vi "一体站流程自动启动.vi"(11 "参数":T1) -> ()   [LabVIEW 2016, in "PLC.lvlib"]
uses:
  PLC.lvlib
  <vilib>/ptbypt/NI_PtbyPt.lvlib
panel:
  out "s? t:f":enum16{"初始化", "采配水启动", "仪器操作", "反冲洗", "结束"}(ring)
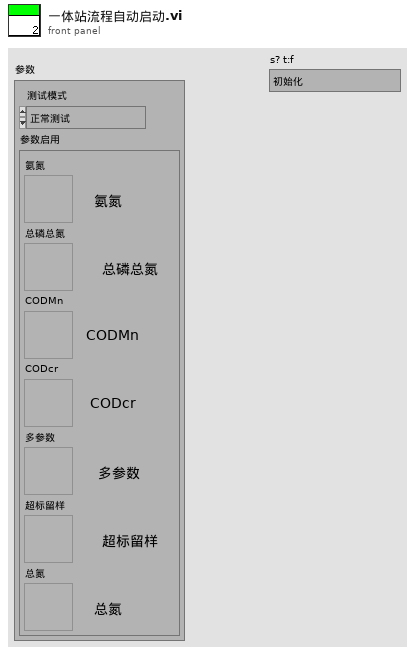
[diagram p1: front panel]
types:
  T1 = cluster{"测试模式":enum16{"正常测试", "集成干预"}, "参数启用":cluster{"氨氮":bool, "总磷总氮":bool, "CODMn":bool, "CODcr":bool, "多参数":bool, "超标留样":bool, "总氮":bool}}
  T2 = cluster{"命令":string, cluster{"starting address":u16, "holding register value":u16}}
  T3 = enum16{"加标流程（润洗/采样分开）", "加标流程（润洗/采样合并）", "加标流程（不启动采配水）", "水样测试（润洗/采样分开）", "水样测试（润洗/采样合并）", "水样测试（不启动采配水）"}
  T4 = typedef "质控单元V4.lvlib/质控slave id.ctl" = enum16{"null", "氨氮", "总磷", "总氮", "CODMn", "CODCr", "氨氮总磷", "总磷总氮"}
  T5 = cluster{"时间标识":timestamp, "设备":string, "日志信息":string, "流程参数":string}
  T6 = cluster{"测量模式":enum16{"水样测量", "标样核查", "零点核查", "跨度核查", "空白测试", "加标回收", "平行样", "校零", "校标"}}
  T7 = cluster{"时间标识":timestamp, "设备":string, "日志信息":string}
  T8 = enum16{"空闲", "水样测试", "标样核查", "零点核查", "跨度核查", "空白测试", "平行样测试", "加标回收", "空白校准", "标样校准", "初始化（清洗）"}
  T9 = enum32{"Bad", "Idle", "Run top level", "Running"}
  T10 = cluster{"R0":i16, "R1":i16, "R2":i16, "R3":i16, "R4":i16, "R5":i16, "R6":i16, "R7":i16, "R8":i16, "R9":i16, "R10":i16, "R11":i16, "R12":i16, "R13":i16, "R14":i16, "R15":i16, "R16":i16, "R17":i16, "R18":i16, "R19":i16, "R20":i16, "R21":i16, "R22":i16, "R23":i16, "R24":i16, "R25":i16, "R26":i16, "R27":i16, "R28":i16, "R29":i16, "R30":i16, "R31":i16, "R32":i16, "R33":i16, "R34":i16, "R35":i16, "R36":i16, "R37":i16, "R38":i16, "R39":i16, "R40":i16, "R41":i16, "R42":i16, "R43":i16, "R44":i16, "R45":i16, "R46":i16, "R47":i16, "R48":i16, "R49":i16, "R50":i16, "R51":i16, "R52":i16, "R53":i16, "R54":i16, "R55":i16, "R56":i16}
  T11 = cluster{"氨氮":bool, "总磷总氮":bool, "CODmn":bool, "CODCr":bool, "多参数":bool, "超标留样":bool, "总氮":bool}
  T12 = cluster{"因子编码":u32, "单位":u16, "标样参考值":sgl, "水样数据时间":timestamp, "水样实测值":sgl, "水样数据标识":string, "标样数据时间":timestamp, "标样实测值":sgl, "标样数据标识":string, "空白数据时间":timestamp, "空白实测值":sgl, "空白数据标识":string, "零点核查数据时间":timestamp, "零点核查实测值":sgl, "零点核查数据标识":string, "跨度核查数据时间":timestamp, "跨度核查实测值":sgl, "跨度核查数据标识":string, "加标回收数据时间":timestamp, "加标回收实测值":sgl, "加标回收数据标识":string, "平行样数据时间":timestamp, "平行样实测值":sgl, "平行样数据标识":string, "F0":sgl, "F1":sgl, "F2":sgl, "F3":sgl, "F4":sgl, "F5":sgl, "F6":sgl, "F7":sgl, "温度":sgl, "湿度":sgl, "X值":sgl, "fidrange":u16}
  T13 = cluster{"COD浓度（mg/L)":dbl, "水样启动时间":timestamp, "加标回收启动时间":timestamp, "CODMn工作状态":enum16{"空闲", "水样测试", "标样核查", "零点核查", "跨度核查", "空白测试", "平行样测试", "加标回收", "空白校准", "标样校准", "初始化（清洗）"}, "多列列表框":i32}
  T14 = cluster{"因子编码":u32, "单位":u16, "标样参考值":sgl, "水样数据时间":timestamp, "水样实测值":sgl, "水样数据标识":string, "标样数据时间":timestamp, "标样实测值":sgl, "标样数据标识":string, "空白数据时间":timestamp, "空白实测值":sgl, "空白数据标识":string, "零点核查数据时间":timestamp, "零点核查实测值":sgl, "零点核查数据标识":string, "跨度核查数据时间":timestamp, "跨度核查实测值":sgl, "跨度核查数据标识":string, "加标回收数据时间":timestamp, "加标回收实测值":sgl, "加标回收数据标识":string, "平行样数据时间":timestamp, "平行样实测值":sgl, "平行样数据标识":string}
  T15 = cluster{"氨氮":bool, "总磷总氮":bool, "CODMn":bool, "CODcr":bool, "多参数":bool, "超标留样":bool, "总氮":bool}
  T16 = cluster{"时间标识":timestamp, "参数":string, "数据类型":string, "集成干预测试浓度值":dbl, "集成干预前测试时间":timestamp, "集成干预前测试浓度值":dbl}
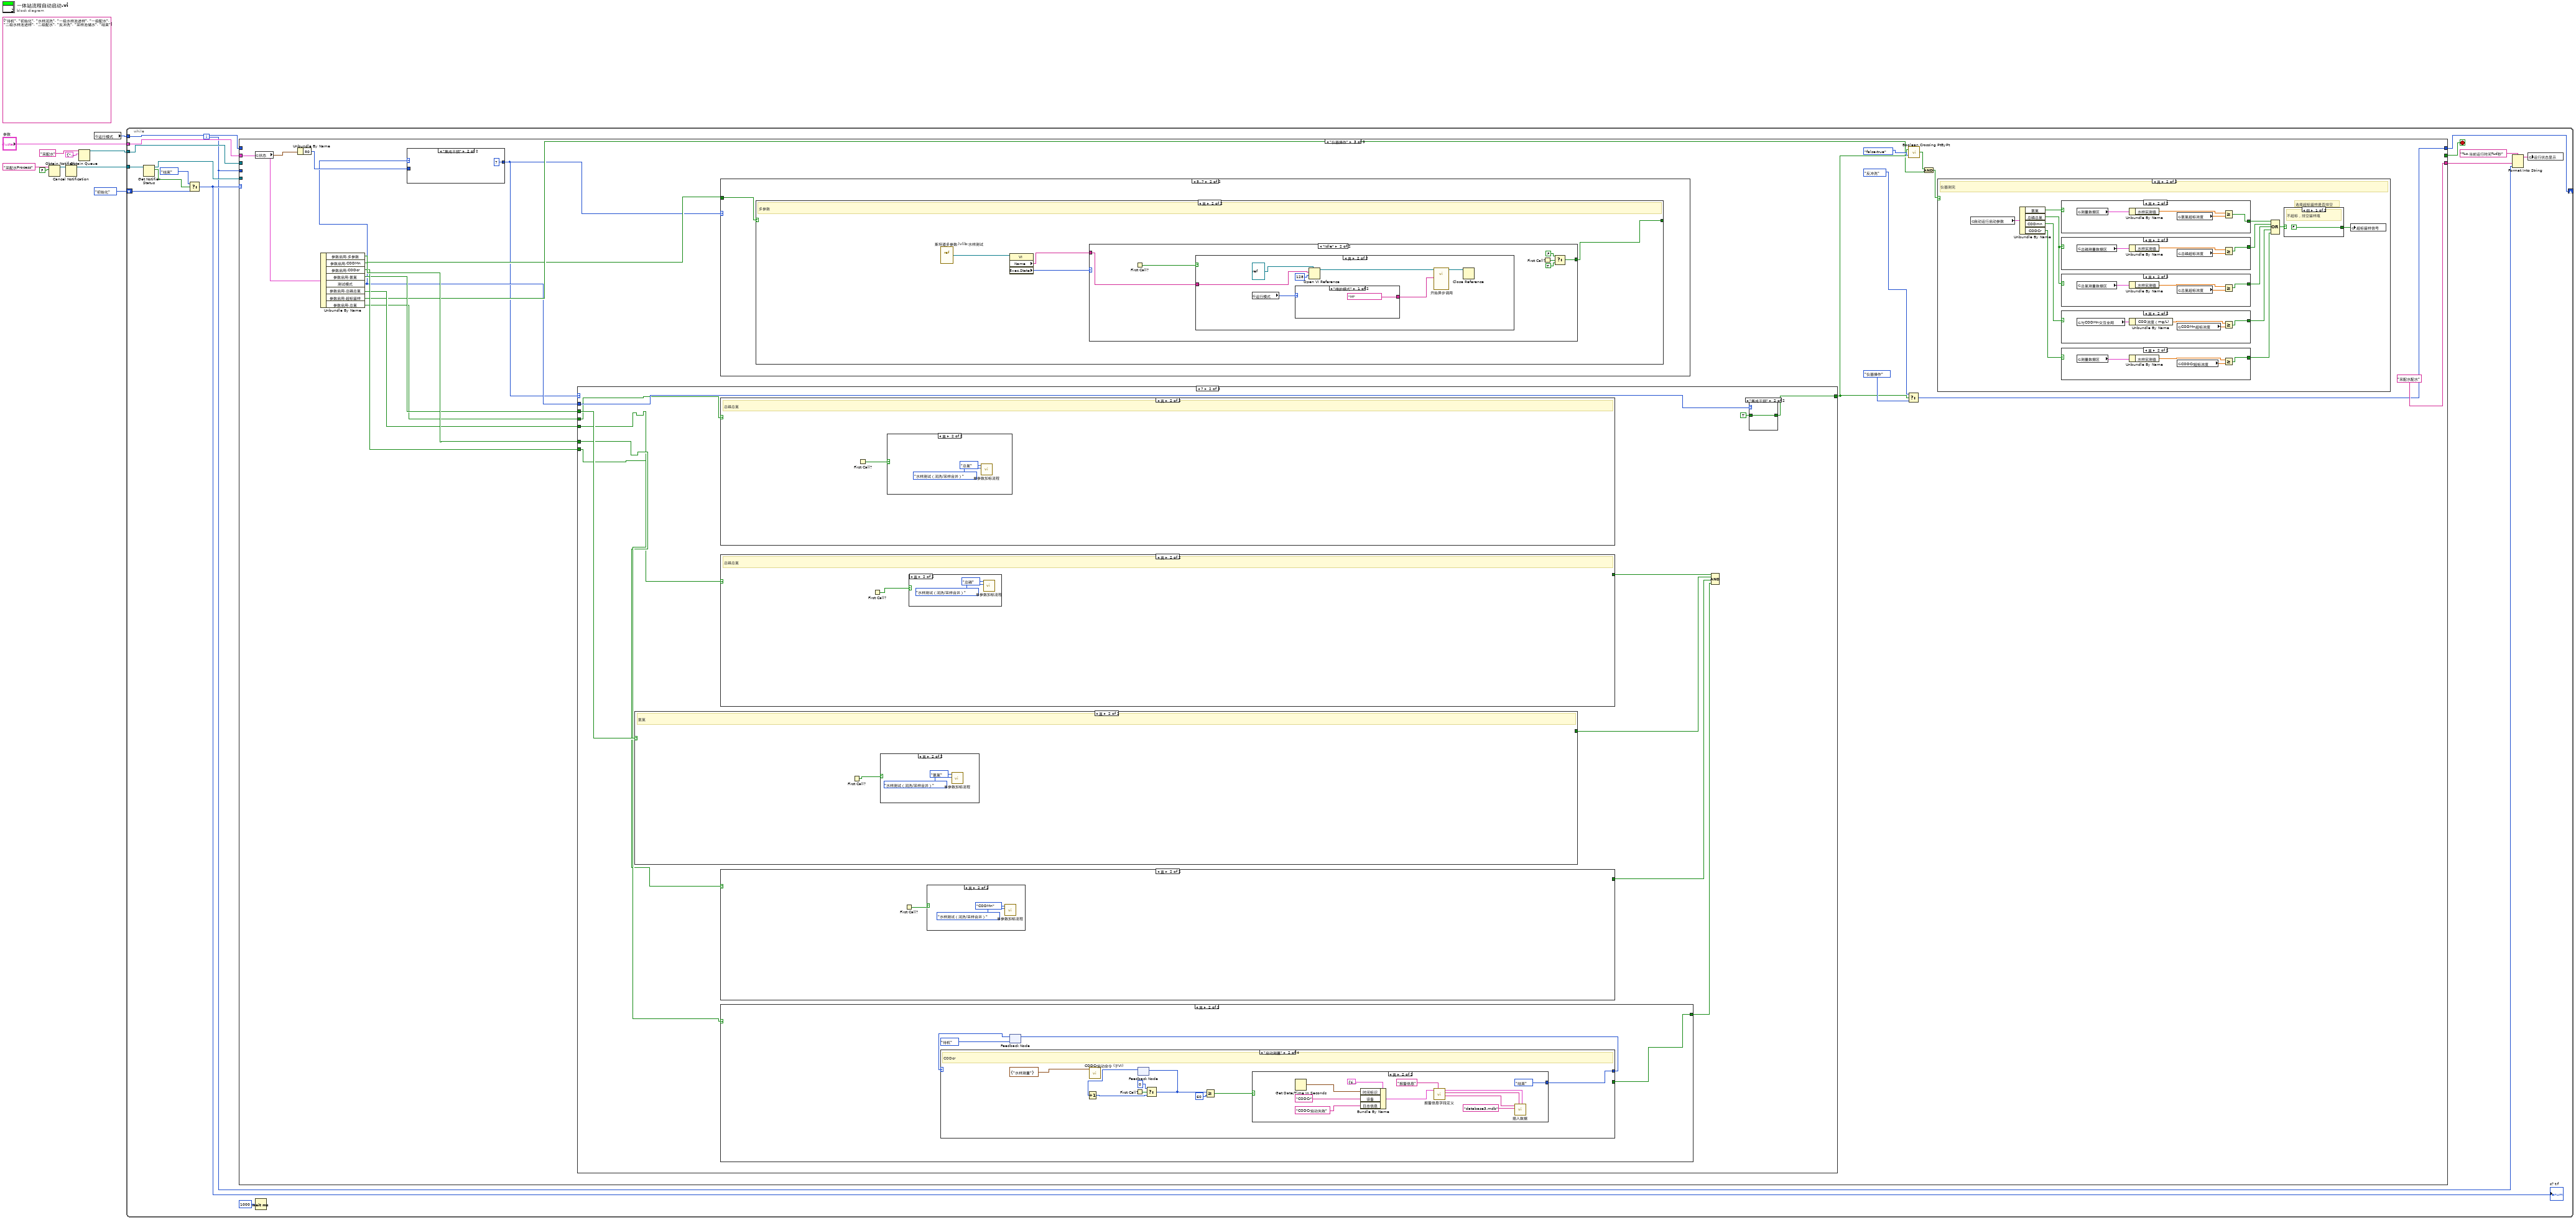
[diagram p0: block diagram]
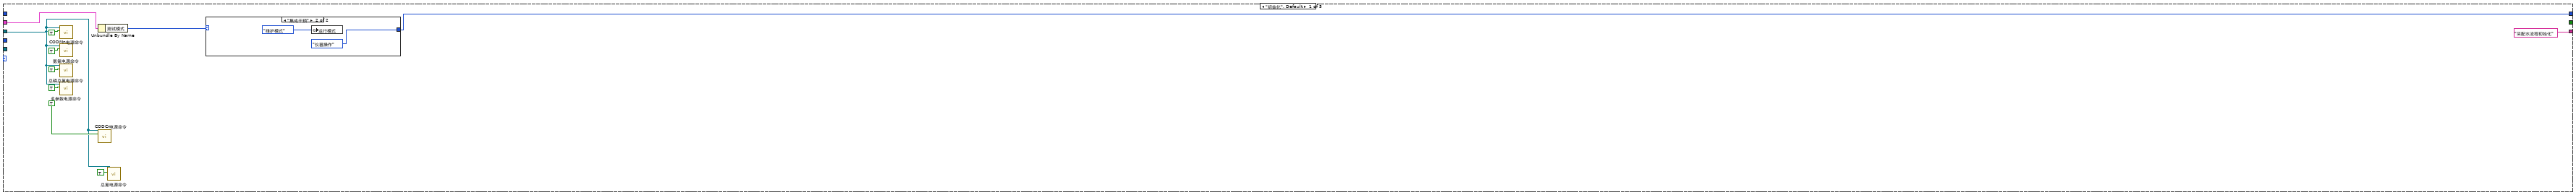
[diagram p2: hidden frame]
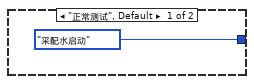
[diagram p3: hidden frame]
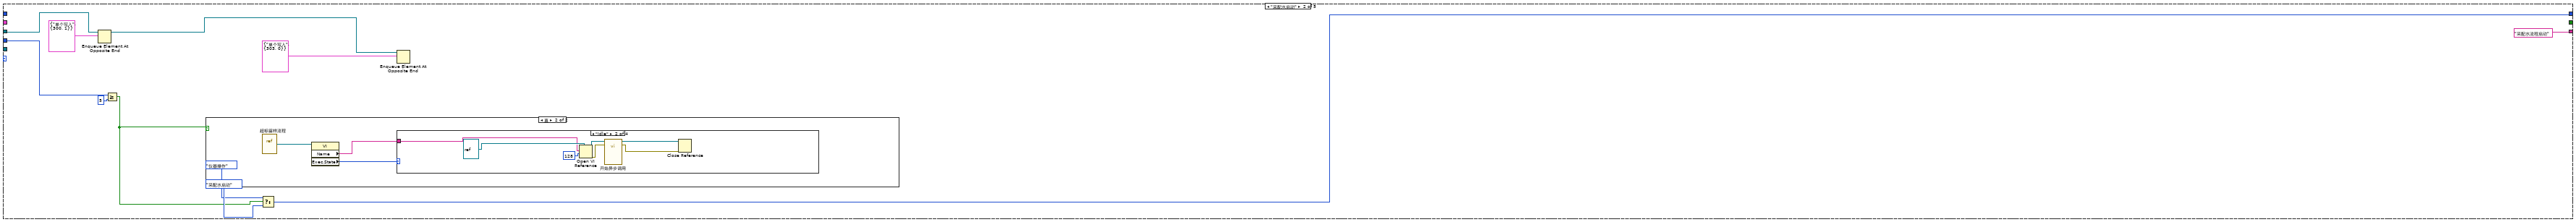
[diagram p4: hidden frame]
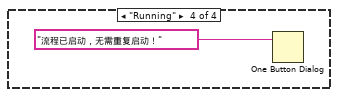
[diagram p8: hidden frame]
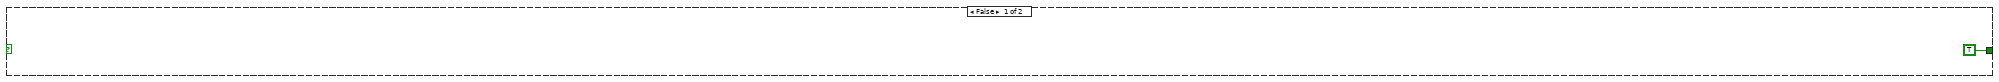
[diagram p10: hidden frame]
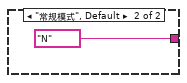
[diagram p13: hidden frame]
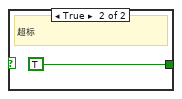
[diagram p15: hidden frame]
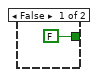
[diagram p16: hidden frame]
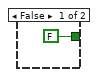
[diagram p17: hidden frame]
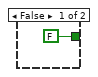
[diagram p18: hidden frame]
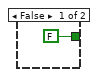
[diagram p19: hidden frame]
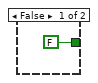
[diagram p20: hidden frame]
diagram:
  (unwired) string[][] [["待机"], ["初始化"], ["水样润洗"], ["一级水样池进样"], ["一级配水"], ["二级水样池进样"], ["二级配水"], ["反冲洗"], ["采样池储水"], ["结束"]] ("项名")
  n1 = Obtain Notifier(name (unnamed)="采配水Process" ("名称（未命名）"), notification data type=FALSE) -> (notifier out=w4:refnum<notifier>)  [unwired: 2 in, 2 out]
  n2 = Cancel Notification(0:w4) -> (8:w3:refnum<notifier>)  [unwired: 1 in, 2 out]
  n3 = Obtain Queue(name (unnamed)="采配水" ("名称（未命名）"), element data type=cluster{"命令":string, "数据":variant} {"命令"="", "数据"=variant}) -> (queue out=w7:refnum<queue>)  [unwired: 3 in, 2 out]
  n4 = global read "系统设置全局变量.vi" "运行模式"() -> (w1:enum16{"维护模式", "常规模式", "应急模式", "质控模式"})
  n5 = while {
    shift-right: [w23] -> _
    shift-left: enum16{"初始化", "采配水启动", "仪器操作", "反冲洗", "结束"}."初始化" ("枚举") -> [w19]
    tunnel: w7 -> [w26]
    tunnel: w3 -> [w22]
    tunnel: "参数" -> [w13]
    tunnel: w1 -> [w12]
    i -> [w11]
    stop <- w25 stop-if-true
    n6 = Get Notifier Status(notifier=w22) -> (notifier out=w14:refnum<notifier>, current notification=w21:bool)  [unwired: 1 in, 3 out]
    n7 = Select(t=enum16{"初始化", "采配水启动", "仪器操作", "反冲洗", "结束"}."结束" ("枚举"), s=w21, f=w19) -> (s? t:f=w18:enum16{"初始化", "采配水启动", "仪器操作", "反冲洗", "结束"})
    "s? t:f" <- w18
    n8 = case shown="\"仪器操作\"" w18 {
      tunnel: w26 -> [w28 w51 _ _ w453]
      tunnel: [_ _ _ _ TRUE] -> w25
      tunnel: [w32 w44 w78 w237 enum16{"初始化", "采配水启动", "仪器操作", "反冲洗", "结束"}."结束" ("枚举")] -> w23
      tunnel: ["采配水流程初始化" "采配水流程启动" "采配水配水" "等待测试完成" "采配水结束"] -> w15
      tunnel: w14 -> [_ _ _ _ w454]
      tunnel: w13 -> [w30 _ w80 w236 w450]
      tunnel: w12 -> [_ _ _ w233 w449]
      tunnel: w11 -> [_ w49 _ _ _]
      frame "初始化", Default {
        n9 = call "CODMn电源命令.vi"("通电/断电"=TRUE, "队列"=w28) -> ()  [unwired: 9 in, 1 out]
        n10 = call "氨氮电源命令.vi"("通电/断电"=TRUE, "队列"=w28) -> ()  [unwired: 9 in, 1 out]
        n11 = call "总磷总氮电源命令.vi"("通电/断电"=TRUE, "队列"=w28) -> ()  [unwired: 9 in, 1 out]
        n12 = call "多参数电源命令.vi"("通电/断电"=TRUE, "队列"=w28) -> ()  [unwired: 9 in, 1 out]
        n13 = Unbundle By Name(w30) -> ("测试模式"=w29:enum16{"正常测试", "集成干预"})
        n14 = call "CODCr电源命令.vi"("通电/断电"=TRUE, "队列"=w28) -> ()  [unwired: 9 in, 1 out]
        n15 = call "总氮电源命令.vi"("通电/断电"=TRUE, "队列"=w28) -> ()  [unwired: 9 in, 1 out]
        n16 = case shown="\"集成干预\"" w29 {
          tunnel: [enum16{"初始化", "采配水启动", "仪器操作", "反冲洗", "结束"}."采配水启动" ("枚举") enum16{"初始化", "采配水启动", "仪器操作", "反冲洗", "结束"}."仪器操作" ("枚举")] -> w32
          frame "正常测试", Default {
          }
          frame "集成干预" {
            n17 = global write "系统设置全局变量.vi" "运行模式"(enum16{"维护模式", "常规模式", "应急模式", "质控模式"}."维护模式" ("运行模式")) -> ()
          }
        }
      }
      frame "采配水启动" {
        n18 = Enqueue Element At Opposite End(queue=w51, element=T2 {"命令"="单个写入", {"starting address"=300, "holding register value"=1}} ("元素")) -> (queue out=w42:refnum<queue>)  [unwired: 2 in, 2 out]
        n19 = Greater Or Equal?(x=w49, y=5) -> (x >= y?=w41:bool)
        n20 = case shown="真" w41 {
          frame False {
          }
          frame True {
            n21 = vi-ref "超标留样流程.vi"() -> (w54:refnum<vi>)
            n22 = property class="VI"(reference=w54) -> ("Name"=w53:string, "Exec.State"=w52:T9)  [unwired: 1 in, 2 out]
            n23 = case shown="\"Idle\"" w52 {
              tunnel: w53 -> [_ w57 _ _]
              frame "Bad", Default {
              }
              frame "Idle" {
                n24 = Open VI Reference(type specifier VI Refnum (for type only)=refnum<vi> refnum ("类型说明符VI引用句柄（仅用于类型）"), vi path=w57, options=128 ("选项")) -> (vi reference=w61:refnum<vi>, error out=w56:errorcluster)  [unwired: 3 in]
                n25 = call-by-ref "开始异步调用"(reference=w61, error in=w56) -> (reference out=w60:refnum<vi>, error out=w55:errorcluster)  [unwired: 12 in]
                n26 = Close Reference(reference=w60, error in (no error)=w55) -> ()  [unwired: 1 out]
              }
              frame "Run top level" {
              }
              frame "Running" {
                n27 = One Button Dialog(message="流程已启动，无需重复启动！" ("消息")) -> ()  [unwired: 1 in, 1 out]
              }
            }
          }
        }
        n28 = Select(t=enum16{"初始化", "采配水启动", "仪器操作", "反冲洗", "结束"}."仪器操作" ("枚举"), s=w41, f=enum16{"初始化", "采配水启动", "仪器操作", "反冲洗", "结束"}."采配水启动" ("枚举")) -> (s? t:f=w44:enum16{"初始化", "采配水启动", "仪器操作", "反冲洗", "结束"})
        n29 = Enqueue Element At Opposite End(queue=w42, element=T2 {"命令"="单个写入", {"starting address"=303, "holding register value"=0}} ("元素")) -> ()  [unwired: 2 in, 3 out]
      }
      frame "仪器操作" {
        n30 = global read "采配水全局变量.vi" "状态"() -> (w82:T10)
        n31 = Unbundle By Name(w82) -> ("R0"=w73:i16)
        n32 = Unbundle By Name(w80) -> ("参数启用.多参数"=w66:bool, "参数启用.CODMn"=w76:bool, "参数启用.CODcr"=w75:bool, "参数启用.氨氮"=w74:bool, "测试模式"=w65:enum16{"正常测试", "集成干预"}, "参数启用.总磷总氮"=w72:bool, "参数启用.超标留样"=w67:bool, "参数启用.总氮"=w64:bool)
        n33 = case shown="\"集成干预\"" w65 {
          tunnel: w73 -> [w143 _]
          tunnel: [w143 i16 7 ("R0")] -> w63
          frame "正常测试", Default {
          }
          frame "集成干预" {
          }
        }
        n34 = case shown="7" w63 {
          tunnel: [w146 w159 TRUE] -> w68
          tunnel: w76 -> [_ w154 _]
          tunnel: w75 -> [_ w155 _]
          tunnel: w74 -> [_ w163 _]
          tunnel: w65 -> [_ w157 _]
          tunnel: w72 -> [_ w153 _]
          tunnel: w64 -> [_ w152 _]
          frame 0, Default {
            n35 = global read "采配水全局变量.vi" "状态"() -> (w149:T10)
            n36 = global read "采配水全局变量.vi" "报警簇"() -> (w150:bool[])
            n37 = Unbundle By Name(w149) -> ("R0"=w148:i16)
            n38 = Index Array(array=w150, index=0 ("索引")) -> (element=w145:bool)
            n39 = Equal To 0?(x=w148) -> (x = 0?=w151:bool)
            n40 = Compound Arithmetic op=OR ("复合运算")(w151, w145) -> (w146:bool)
          }
          frame 7 {
            n41 = case "条件结构" shown="真" w163 {
              tunnel: [TRUE ("t") _] -> w162
              frame False {
              }
              frame True {
                # "氨氮"
                n42 = First Call?() -> (First Call?: T/F=w173:bool)
                n43 = case shown="真" w173 {
                  frame False {
                  }
                  frame True {
                    n44 = call "单参数加标流程.vi"("流程类型"=T3."水样测试（润洗/采样合并）", "Slave ID"=质控slave_id."氨氮") -> ()  [unwired: 10 in]
                  }
                }
              }
            }
            n45 = case "条件结构" shown="真" w152 {
              frame False {
                (unwired) TRUE ("t")
              }
              frame True {
                # "总磷总氮"
                n46 = First Call?() -> (First Call?: T/F=w164:bool)
                n47 = case shown="真" w164 {
                  frame False {
                  }
                  frame True {
                    n48 = call "单参数加标流程.vi"("流程类型"=T3."水样测试（润洗/采样合并）", "Slave ID"=质控slave_id."总氮") -> ()  [unwired: 10 in]
                  }
                }
              }
            }
            n49 = case "条件结构" shown="真" w153 {
              tunnel: [TRUE ("t") _] -> w158
              frame False {
              }
              frame True {
                # "总磷总氮"
                n50 = First Call?() -> (First Call?: T/F=w168:bool)
                n51 = case shown="真" w168 {
                  frame False {
                  }
                  frame True {
                    n52 = call "单参数加标流程.vi"("流程类型"=T3."水样测试（润洗/采样合并）", "Slave ID"=质控slave_id."总磷") -> ()  [unwired: 10 in]
                  }
                }
              }
            }
            n53 = case shown="真" w154 {
              tunnel: [TRUE _] -> w161
              frame False {
              }
              frame True {
                n54 = First Call?() -> (First Call?: T/F=w229:bool)
                n55 = case shown="真" w229 {
                  frame False {
                  }
                  frame True {
                    n56 = call "单参数加标流程.vi"("流程类型"=T3."水样测试（润洗/采样合并）", "Slave ID"=质控slave_id."CODMn") -> ()  [unwired: 10 in]
                  }
                }
              }
            }
            n57 = case shown="真" w155 {
              tunnel: [TRUE w180] -> w160
              frame False {
              }
              frame True {
                n58 = feedback #1(enum16{"待机", "启动测量", "测量中", "结束"}."待机") -> (w178:enum16{"待机", "启动测量", "测量中", "结束"})
                n59 = case shown="\"启动测量\"" w178 {
                  tunnel: [enum16{"待机", "启动测量", "测量中", "结束"}."启动测量" w195 w215 enum16{"待机", "启动测量", "测量中", "结束"}."结束"] -> w177
                  tunnel: [_ _ _ TRUE] -> w180
                  frame "待机", Default {
                    n60 = Get Date/Time In Seconds() -> (seconds since 1Jan1904=w185:timestamp)
                    n61 = Bundle By Name(cluster=T5 {"时间标识"=timestamp(0 s since 1904-01-01), "设备"="", "日志信息"="", "流程参数"=""} ("data in"), "时间标识"=w185, "设备"="CODCr", "日志信息"="-->>CODCr启动") -> (w181:T5)
                    n62 = call "总磷总氮操作日志.vi"("data in"=w181) -> ()  [unwired: 11 in]
                  }
                  frame "启动测量" {
                    # "CODcr"
                    n63 = call "CODCr启动命令 (子VI).vi"("启动测量模式"=T6 {"测量模式"=enum."水样测量"}) -> ()  [unwired: 11 in]
                    n64 = First Call?() -> (First Call?: T/F=w190:bool)
                    n65 = feedback #2() -> (w191:i32)  [unwired: 1 in]
                    n66 = Increment(x=w191) -> (x+1=w192:i32)
                    n67 = Select(t=0, s=w190, f=w192) -> (s? t:f=w193:i32)
                    n68 = feedback-in #2(w193) -> ()
                    n69 = Greater Or Equal?(x=w193, y=60) -> (x >= y?=w188:bool)
                    n70 = case shown="真" w188 {
                      tunnel: [w196 enum16{"待机", "启动测量", "测量中", "结束"}."结束"] -> w195
                      frame False {
                        n71 = global read "CODcr全局变量.vi" "工作状态"() -> (w197:T8)
                        n72 = Not Equal To 0?(x=w197) -> (x != 0?=w198:bool)
                        n73 = Select(t=enum16{"待机", "启动测量", "测量中", "结束"}."测量中", s=w198, f=enum16{"待机", "启动测量", "测量中", "结束"}."启动测量") -> (s? t:f=w196:enum16{"待机", "启动测量", "测量中", "结束"})
                      }
                      frame True {
                        n74 = Get Date/Time In Seconds() -> (seconds since 1Jan1904=w207:timestamp)
                        n75 = Bundle By Name(cluster=T7 {"时间标识"=timestamp(0 s since 1904-01-01), "设备"="", "日志信息"=""} ("data in"), "时间标识"=w207, "设备"="CODCr", "日志信息"="CODCr启动失败") -> (w201:T7)
                        n76 = call "报警信息字段定义.vi"("table输入"="报警信息", "data in"=w201) -> ("table输出"=w204:string, "columns"=w205:string[], "data out"=w206:T7)  [unwired: 7 in]
                        n77 = call "插入数据.vi"("data"=w206, "columns"=w205, "database"="database3.mdb", "table"=w204) -> ()  [unwired: 7 in, 1 out]
                      }
                    }
                  }
                  frame "测量中" {
                    n78 = global read "CODcr全局变量.vi" "工作状态"() -> (w214:T8)
                    n79 = Equal?(x=w214, y=T8."空闲" ("工作状态")) -> (x = y?=w213:bool)
                    n80 = case shown="假" w213 {
                      tunnel: [w216 enum16{"待机", "启动测量", "测量中", "结束"}."结束"] -> w215
                      frame False {
                        n81 = flat-sequence {
                          tunnel: [enum16{"待机", "启动测量", "测量中", "结束"}."测量中"] -> w216
                          frame #0 {
                            n82 = Wait (ms)(milliseconds to wait=u32 1000 ("等待时间（毫秒）")) -> ()  [unwired: 1 out]
                          }
                          frame #1 {
                          }
                        }
                      }
                      frame True {
                      }
                    }
                  }
                  frame "结束" {
                    n83 = First Call?() -> (First Call?: T/F=w220:bool)
                    n84 = case shown="真" w220 {
                      frame False {
                      }
                      frame True {
                        n85 = Get Date/Time In Seconds() -> (seconds since 1Jan1904=w227:timestamp)
                        n86 = Bundle By Name(cluster=T5 {"时间标识"=timestamp(0 s since 1904-01-01), "设备"="", "日志信息"="", "流程参数"=""} ("data in"), "时间标识"=w227, "设备"="CODCr", "日志信息"="-->>CODCr停止") -> (w223:T5)
                        n87 = call "总磷总氮操作日志.vi"("data in"=w223) -> ()  [unwired: 11 in]
                      }
                    }
                  }
                }
                n88 = feedback-in #1(w177) -> ()
              }
            }
            n89 = Compound Arithmetic op=AND ("复合运算")(w158, w162, w161, w160) -> ()  [unwired: 1 out]
            n90 = case shown="\"集成干预\"" w157 {
              tunnel: TRUE -> [_ w171]
              tunnel: [_ w171] -> w159
              frame "正常测试", Default {
              }
              frame "集成干预" {
              }
            }
          }
          frame 8, 9 {
          }
        }
        n91 = case shown="5..7" w63 {
          tunnel: w66 -> [_ w83]
          frame 0, Default {
          }
          frame 5..7 {
            n92 = case shown="真" w83 {
              tunnel: [TRUE ("t") w88] -> _
              frame False {
              }
              frame True {
                # "多参数"
                n93 = vi-ref "斯坦道多参数.lvlib:水样测试.vi"() -> (w86:refnum<vi>)
                n94 = property class="VI"(reference=w86) -> ("Name"=w85:string, "Exec.State"=w87:T9)  [unwired: 1 in, 2 out]
                n95 = case shown="\"Idle\"" w87 {
                  tunnel: w85 -> [_ w94]
                  tunnel: [_ w89] -> w88
                  frame "Bad", Default {
                  }
                  frame "Idle" {
                    n96 = First Call?() -> (First Call?: T/F=w93:bool)
                    n97 = case shown="真" w93 {
                      tunnel: w94 -> [_ w100]
                      frame False {
                      }
                      frame True {
                        n98 = global read "系统设置全局变量.vi" "运行模式"() -> (w97:enum16{"维护模式", "常规模式", "应急模式", "质控模式"})
                        n99 = case shown="\"维护模式\"" w97 {
                          tunnel: ["M" ("数据标记表") "N" ("数据标记表")] -> w96
                          frame "维护模式" {
                          }
                          frame "常规模式", Default {
                          }
                        }
                        n100 = Open VI Reference(type specifier VI Refnum (for type only)=refnum<vi> refnum, vi path=w100, options=128 ("选项")) -> (vi reference=w99:refnum<vi>)  [unwired: 3 in, 1 out]
                        n101 = call-by-ref "开始异步调用"(reference=w99, "数据标记表"=w96) -> (reference out=w98:refnum<vi>)  [unwired: 12 in, 1 out]
                        n102 = Close Reference(reference=w98) -> ()  [unwired: 1 in, 1 out]
                      }
                    }
                    n103 = First Call?() -> (First Call?: T/F=w92:bool)
                    n104 = Select(t=FALSE, s=w92, f=TRUE) -> (s? t:f=w89:bool)
                  }
                }
              }
            }
          }
        }
        n105 = Select(t=enum16{"初始化", "采配水启动", "仪器操作", "反冲洗", "结束"}."反冲洗" ("枚举"), s=w68, f=enum16{"初始化", "采配水启动", "仪器操作", "反冲洗", "结束"}."仪器操作" ("枚举")) -> (s? t:f=w78:enum16{"初始化", "采配水启动", "仪器操作", "反冲洗", "结束"})
        n106 = call <vilib>:"Boolean Crossing PtByPt.vi"("direction"=enum16{"either", "false-true", "true-false"}."false-true", "input"=w68) -> ("crossing"=w70:bool)  [unwired: 1 in]
        n107 = And(x=w70, y=w67) -> (x .and. y?=w69:bool)
        n108 = case shown="真" w69 {
          frame False {
          }
          frame True {
            # "选择超标留样是否排空"
            # "仪器测完"
            n109 = global read "系统设置全局变量.vi" "自动运行启动参数"() -> (w108:T11)
            n110 = Unbundle By Name(w108) -> ("氨氮"=w107:bool, "总磷总氮"=w106:bool, "CODmn"=w105:bool, "CODCr"=w104:bool)
            n111 = case shown="真" w107 {
              tunnel: [FALSE w141] -> w115
              frame False {
              }
              frame True {
                n112 = global read "VAR总磷总氮全局变量.vi" "测量数据区"() -> (w140:T12)
                n113 = Unbundle By Name(w140) -> ("水样实测值"=w142:sgl)
                n114 = global read "外部交互全局.vi" "氨氮超标浓度"() -> (w139:dbl)
                n115 = Greater Or Equal?(x=w142, y=w139) -> (x >= y?=w141:bool)
              }
            }
            n116 = case shown="真" w106 {
              tunnel: [FALSE w137] -> w114
              frame False {
              }
              frame True {
                n117 = global read "VAR总磷总氮全局变量.vi" "总磷测量数据区"() -> (w134:T12)
                n118 = Unbundle By Name(w134) -> ("水样实测值"=w136:sgl)
                n119 = global read "外部交互全局.vi" "总磷超标浓度"() -> (w135:dbl)
                n120 = Greater Or Equal?(x=w136, y=w135) -> (x >= y?=w137:bool)
              }
            }
            n121 = case shown="真" w106 {
              tunnel: [FALSE w132] -> w113
              frame False {
              }
              frame True {
                n122 = global read "VAR总磷总氮全局变量.vi" "总氮测量数据区"() -> (w129:T12)
                n123 = Unbundle By Name(w129) -> ("水样实测值"=w131:sgl)
                n124 = global read "外部交互全局.vi" "总氮超标浓度"() -> (w130:dbl)
                n125 = Greater Or Equal?(x=w131, y=w130) -> (x >= y?=w132:bool)
              }
            }
            n126 = case shown="真" w105 {
              tunnel: [FALSE w127] -> w112
              frame False {
              }
              frame True {
                n127 = global read "modbus slave全局.vi" "与CODMn交互全局"() -> (w125:T13)
                n128 = Unbundle By Name(w125) -> ("COD浓度（mg/L)"=w124:dbl)
                n129 = global read "外部交互全局.vi" "CODMn超标浓度"() -> (w126:dbl)
                n130 = Greater Or Equal?(x=w124, y=w126) -> (x >= y?=w127:bool)
              }
            }
            n131 = case shown="真" w104 {
              tunnel: [FALSE w122] -> w111
              frame False {
              }
              frame True {
                n132 = global read "CODcr全局变量.vi" "测量数据区"() -> (w119:T14)
                n133 = Unbundle By Name(w119) -> ("水样实测值"=w121:sgl)
                n134 = global read "外部交互全局.vi" "CODCr超标浓度"() -> (w120:dbl)
                n135 = Greater Or Equal?(x=w121, y=w120) -> (x >= y?=w122:bool)
              }
            }
            n136 = Compound Arithmetic op=OR ("复合运算")(w115, w114, w113, w112, w111) -> (w110:bool)
            n137 = case shown="假" w110 {
              tunnel: [FALSE ("超标留样信号") TRUE ("超标留样信号")] -> w109
              frame False {
                # "不超标，排空留样瓶"
              }
              frame True {
                # "超标"
              }
            }
            n138 = global write "外部交互全局.vi" "超标留样信号"(w109) -> ()
          }
        }
      }
      frame "反冲洗" {
        n139 = First Call?() -> (First Call?: T/F=w234:bool)
        n140 = global read "采配水全局变量.vi" "状态"() -> (w242:T10)
        n141 = case shown="真" w234 {
          tunnel: w236 -> [_ w246]
          tunnel: w233 -> [_ w243]
          frame False {
          }
          frame True {
            n142 = Unbundle By Name(w246) -> ("测试模式"=w245:enum16{"正常测试", "集成干预"}, "参数启用"=w244:T15)
            n143 = case shown="\"正常测试\", 默认" w245 {
              tunnel: w244 -> [w255 w366]
              tunnel: w243 -> [_ w360]
              frame "正常测试", Default {
                n144 = global read "系统设置全局变量.vi" "运行模式"() -> (w253:enum16{"维护模式", "常规模式", "应急模式", "质控模式"})
                n145 = global read "采配水全局变量.vi" "报警簇"() -> (w260:bool[])
                n146 = global read "采配水全局变量.vi" "输入状态"() -> (w252:bool[])
                n147 = case shown="\"维护模式\"" w253 {
                  tunnel: ["M" ("table") "N" ("table")] -> w254
                  frame "维护模式" {
                  }
                  frame "常规模式", Default {
                  }
                }
                n148 = Index Array(array=w252, index=7 ("索引")) -> (element=w250:bool)
                n149 = Index Array(array=w260, index #1=0 ("索引"), index #2=11 ("索引")) -> (element #1=w257:bool, element #2=w256:bool)
                n150 = Select(t="P" ("数据标识"), s=w250, f="Z" ("数据标识")) -> (s? t:f=w247:string)
                n151 = case shown="真" w257 {
                  tunnel: w256 -> [w266 w274]
                  tunnel: w255 -> [w265 w284]
                  tunnel: w254 -> [w263 w277]
                  tunnel: w247 -> [_ w276]
                  frame False {
                    n152 = Unbundle By Name(w265) -> ("氨氮"=w264:bool)
                    n153 = case shown="真" w266 {
                      tunnel: w264 -> [_ w268]
                      tunnel: w263 -> [_ w267]
                      frame False {
                      }
                      frame True {
                        n154 = case shown="真" w268 {
                          tunnel: w267 -> [_ w269]
                          tunnel: [_ w270] -> _
                          frame False {
                          }
                          frame True {
                            n155 = call "取水点无水样数据存储.vi"("数据标识"="lw", "数据类型"=w269, "table"="氨氮") -> ("error out"=w270:errorcluster)  [unwired: 8 in]
                          }
                        }
                      }
                    }
                  }
                  frame True {
                    n156 = Unbundle By Name(w284) -> ("氨氮"=w283:bool, "CODMn"=w282:bool, "CODcr"=w281:bool, "多参数"=w280:bool, "总磷总氮"=w279:bool, "总氮"=w278:bool)
                    n157 = Not(x=w274) -> (.not. x?=w273:bool)
                    n158 = And(x=w280, y=w273) -> (x .and. y?=w275:bool)
                    n159 = case shown="真" w283 {
                      tunnel: w277 -> [_ w351]
                      tunnel: w276 -> [_ w350]
                      tunnel: [_ w349] -> _
                      frame False {
                      }
                      frame True {
                        n160 = global read "系统设置全局变量.vi" "营养盐类型"() -> (w348:enum16{"氨氮、总磷总氮", "氨氮总磷", "氨氮、总磷、总氮"})
                        n161 = call "取水点无水样数据存储.vi"("数据标识"=w350, "数据类型"=w351, "table"="氨氮") -> ("error out"=w352:errorcluster)  [unwired: 8 in]
                        n162 = case shown="\"氨氮总磷\"" w348 {
                          tunnel: w352 -> [_ w357]
                          tunnel: w351 -> [_ w356]
                          tunnel: w350 -> [_ w355]
                          tunnel: [_ w354] -> w349
                          frame "氨氮、总磷总氮", Default {
                          }
                          frame "氨氮总磷" {
                            n163 = call "取水点无水样数据存储.vi"("error in (no error)"=w357, "数据标识"=w355, "数据类型"=w356, "table"="总磷") -> ("error out"=w354:errorcluster)  [unwired: 7 in]
                          }
                        }
                      }
                    }
                    n164 = case shown="真" w278 {
                      tunnel: w277 -> [_ w287]
                      tunnel: w276 -> [_ w288]
                      tunnel: [_ w286] -> _
                      frame False {
                      }
                      frame True {
                        n165 = global read "系统设置全局变量.vi" "营养盐类型"() -> (w285:enum16{"氨氮、总磷总氮", "氨氮总磷", "氨氮、总磷、总氮"})
                        n166 = case shown="\"氨氮、总磷、总氮\"" w285 {
                          tunnel: w288 -> [_ w291]
                          tunnel: w287 -> [_ w290]
                          tunnel: [_ w289] -> w286
                          frame "氨氮、总磷总氮", Default {
                          }
                          frame "氨氮、总磷、总氮" {
                            n167 = call "取水点无水样数据存储.vi"("数据标识"=w291, "数据类型"=w290, "table"="总氮") -> ("error out"=w289:errorcluster)  [unwired: 8 in]
                          }
                        }
                      }
                    }
                    n168 = case shown="真" w282 {
                      tunnel: w277 -> [_ w346]
                      tunnel: [_ w345] -> _
                      tunnel: w276 -> [_ w344]
                      frame False {
                      }
                      frame True {
                        n169 = call "取水点无水样数据存储.vi"("数据标识"=w344, "数据类型"=w346, "table"="CODMn") -> ("error out"=w345:errorcluster)  [unwired: 8 in]
                      }
                    }
                    n170 = case shown="真" w281 {
                      tunnel: w277 -> [_ w342]
                      tunnel: [_ w341] -> _
                      tunnel: w276 -> [_ w340]
                      frame False {
                      }
                      frame True {
                        n171 = call "取水点无水样数据存储.vi"("数据标识"=w340, "数据类型"=w342, "table"="CODCr") -> ("error out"=w341:errorcluster)  [unwired: 8 in]
                      }
                    }
                    n172 = case shown="真" w279 {
                      tunnel: w277 -> [_ w295]
                      tunnel: [_ w296] -> _
                      tunnel: w276 -> [_ w294]
                      frame False {
                      }
                      frame True {
                        n173 = global read "系统设置全局变量.vi" "营养盐类型"() -> (w293:enum16{"氨氮、总磷总氮", "氨氮总磷", "氨氮、总磷、总氮"})
                        n174 = case shown="\"氨氮总磷\", 默认" w293 {
                          tunnel: [w301 _] -> w297
                          tunnel: w294 -> [w300 _]
                          tunnel: w295 -> [w299 _]
                          frame "氨氮、总磷总氮" {
                            n175 = call "取水点无水样数据存储.vi"("数据标识"=w300, "数据类型"=w299, "table"="总氮") -> ("error out"=w301:errorcluster)  [unwired: 8 in]
                          }
                          frame "氨氮总磷", Default {
                          }
                        }
                        n176 = call "取水点无水样数据存储.vi"("error in (no error)"=w297, "数据标识"=w294, "数据类型"=w295, "table"="总磷") -> ("error out"=w296:errorcluster)  [unwired: 7 in]
                      }
                    }
                    n177 = case shown="真" w275 {
                      tunnel: w277 -> [_ w311]
                      tunnel: w276 -> [_ w303]
                      frame False {
                      }
                      frame True {
                        n178 = global read "断电保存变量.vi" "pH"() -> (w309:bool)
                        n179 = global read "断电保存变量.vi" "DO"() -> (w308:bool)
                        n180 = global read "断电保存变量.vi" "Turb"() -> (w307:bool)
                        n181 = global read "断电保存变量.vi" "Temp"() -> (w310:bool)
                        n182 = global read "断电保存变量.vi" "Cond"() -> (w306:bool)
                        n183 = global read "断电保存变量.vi" "藻密度"() -> (w304:bool)
                        n184 = global read "断电保存变量.vi" "叶绿素a启用"() -> (w305:bool)
                        n185 = case shown="真" w309 {
                          tunnel: w311 -> [_ w334]
                          tunnel: [_ w333] -> _
                          tunnel: w303 -> [_ w332]
                          frame False {
                          }
                          frame True {
                            n186 = call "取水点无水样数据存储.vi"("数据标识"=w332, "数据类型"=w334, "table"="pH") -> ("error out"=w333:errorcluster)  [unwired: 8 in]
                          }
                        }
                        n187 = case shown="真" w308 {
                          tunnel: w311 -> [_ w330]
                          tunnel: [_ w329] -> _
                          tunnel: w303 -> [_ w328]
                          frame False {
                          }
                          frame True {
                            n188 = call "取水点无水样数据存储.vi"("数据标识"=w328, "数据类型"=w330, "table"="DO") -> ("error out"=w329:errorcluster)  [unwired: 8 in]
                          }
                        }
                        n189 = case shown="真" w307 {
                          tunnel: w311 -> [_ w322]
                          tunnel: [_ w321] -> _
                          tunnel: w303 -> [_ w320]
                          frame False {
                          }
                          frame True {
                            n190 = call "取水点无水样数据存储.vi"("数据标识"=w320, "数据类型"=w322, "table"="浊度") -> ("error out"=w321:errorcluster)  [unwired: 8 in]
                          }
                        }
                        n191 = case shown="真" w310 {
                          tunnel: w311 -> [_ w338]
                          tunnel: [_ w337] -> _
                          tunnel: w303 -> [_ w336]
                          frame False {
                          }
                          frame True {
                            n192 = call "取水点无水样数据存储.vi"("数据标识"=w336, "数据类型"=w338, "table"="水温") -> ("error out"=w337:errorcluster)  [unwired: 8 in]
                          }
                        }
                        n193 = case shown="真" w306 {
                          tunnel: w311 -> [_ w326]
                          tunnel: [_ w325] -> _
                          tunnel: w303 -> [_ w324]
                          frame False {
                          }
                          frame True {
                            n194 = call "取水点无水样数据存储.vi"("数据标识"=w324, "数据类型"=w326, "table"="电导率") -> ("error out"=w325:errorcluster)  [unwired: 8 in]
                          }
                        }
                        n195 = case shown="真" w304 {
                          tunnel: w311 -> [_ w314]
                          tunnel: [_ w313] -> _
                          tunnel: w303 -> [_ w312]
                          frame False {
                          }
                          frame True {
                            n196 = call "取水点无水样数据存储.vi"("数据标识"=w312, "数据类型"=w314, "table"="藻密度") -> ("error out"=w313:errorcluster)  [unwired: 8 in]
                          }
                        }
                        n197 = case shown="真" w305 {
                          tunnel: w311 -> [_ w318]
                          tunnel: [_ w317] -> _
                          tunnel: w303 -> [_ w316]
                          frame False {
                          }
                          frame True {
                            n198 = call "取水点无水样数据存储.vi"("数据标识"=w316, "数据类型"=w318, "table"="叶绿素a") -> ("error out"=w317:errorcluster)  [unwired: 8 in]
                          }
                        }
                      }
                    }
                  }
                }
              }
              frame "集成干预" {
                n199 = Unbundle By Name(w366) -> ("氨氮"=w365:bool, "CODMn"=w364:bool, "CODcr"=w363:bool, "多参数"=w362:bool, "总磷总氮"=w361:bool, "总氮"=w359:bool)
                n200 = case shown="真" w365 {
                  tunnel: w360 -> [_ w445]
                  frame False {
                  }
                  frame True {
                    n201 = call "获取最近两组水样测试数据.vi"("运行模式"=w445, "table"="氨氮") -> ("error out"=w446:errorcluster, "存储变量"=w447:T16)  [unwired: 8 in]
                    n202 = call "集成干预测试数据存储.vi"("error in (no error)"=w446, "存储变量"=w447) -> ()  [unwired: 9 in, 1 out]
                  }
                }
                n203 = case shown="真" w359 {
                  tunnel: w360 -> [_ w367]
                  frame False {
                  }
                  frame True {
                    n204 = call "获取最近两组水样测试数据.vi"("运行模式"=w367, "table"="总氮") -> ("error out"=w370:errorcluster, "存储变量"=w369:T16)  [unwired: 8 in]
                    n205 = call "集成干预测试数据存储.vi"("error in (no error)"=w370, "存储变量"=w369) -> ()  [unwired: 9 in, 1 out]
                  }
                }
                n206 = case shown="真" w364 {
                  tunnel: w360 -> [_ w441]
                  frame False {
                  }
                  frame True {
                    n207 = call "获取最近两组水样测试数据.vi"("运行模式"=w441, "table"="CODMn") -> ("error out"=w442:errorcluster, "存储变量"=w443:T16)  [unwired: 8 in]
                    n208 = call "集成干预测试数据存储.vi"("error in (no error)"=w442, "存储变量"=w443) -> ()  [unwired: 9 in, 1 out]
                  }
                }
                n209 = case shown="真" w363 {
                  tunnel: w360 -> [_ w437]
                  frame False {
                  }
                  frame True {
                    n210 = call "获取最近两组水样测试数据.vi"("运行模式"=w437, "table"="CODCr") -> ("error out"=w438:errorcluster, "存储变量"=w439:T16)  [unwired: 8 in]
                    n211 = call "集成干预测试数据存储.vi"("error in (no error)"=w438, "存储变量"=w439) -> ()  [unwired: 9 in, 1 out]
                  }
                }
                n212 = case shown="真" w361 {
                  tunnel: w360 -> [_ w372]
                  frame False {
                  }
                  frame True {
                    n213 = call "获取最近两组水样测试数据.vi"("运行模式"=w372, "table"="总磷") -> ("error out"=w374:errorcluster, "存储变量"=w375:T16)  [unwired: 8 in]
                    n214 = call "集成干预测试数据存储.vi"("error in (no error)"=w374, "存储变量"=w375) -> ("error out"=w373:errorcluster)  [unwired: 9 in]
                    n215 = global read "系统设置全局变量.vi" "总氮启用"() -> (w371:bool)
                    n216 = case shown="真" w371 {
                      tunnel: w373 -> [_ w378]
                      tunnel: w372 -> [_ w377]
                      frame False {
                      }
                      frame True {
                        n217 = call "获取最近两组水样测试数据.vi"("error in (no error)"=w378, "运行模式"=w377, "table"="总氮") -> ("error out"=w381:errorcluster, "存储变量"=w380:T16)  [unwired: 7 in]
                        n218 = call "集成干预测试数据存储.vi"("error in (no error)"=w381, "存储变量"=w380) -> ()  [unwired: 9 in, 1 out]
                      }
                    }
                  }
                }
                n219 = case shown="真" w362 {
                  tunnel: w360 -> [_ w382]
                  frame False {
                  }
                  frame True {
                    n220 = global read "断电保存变量.vi" "Temp"() -> (w389:bool)
                    n221 = case shown="真" w389 {
                      tunnel: [_ w433] -> w395
                      tunnel: w382 -> [_ w432]
                      frame False {
                      }
                      frame True {
                        n222 = call "获取最近两组水样测试数据.vi"("运行模式"=w432, "table"="水温") -> ("error out"=w436:errorcluster, "存储变量"=w435:T16)  [unwired: 8 in]
                        n223 = call "集成干预测试数据存储.vi"("error in (no error)"=w436, "存储变量"=w435) -> ("error out"=w433:errorcluster)  [unwired: 9 in]
                      }
                    }
                    n224 = global read "断电保存变量.vi" "pH"() -> (w388:bool)
                    n225 = case shown="真" w388 {
                      tunnel: [_ w428] -> w394
                      tunnel: w395 -> [_ w427]
                      tunnel: w382 -> [_ w426]
                      frame False {
                      }
                      frame True {
                        n226 = call "获取最近两组水样测试数据.vi"("error in (no error)"=w427, "运行模式"=w426, "table"="pH") -> ("error out"=w431:errorcluster, "存储变量"=w430:T16)  [unwired: 7 in]
                        n227 = call "集成干预测试数据存储.vi"("error in (no error)"=w431, "存储变量"=w430) -> ("error out"=w428:errorcluster)  [unwired: 9 in]
                      }
                    }
                    n228 = global read "断电保存变量.vi" "DO"() -> (w387:bool)
                    n229 = case shown="真" w387 {
                      tunnel: [_ w422] -> w393
                      tunnel: w394 -> [_ w421]
                      tunnel: w382 -> [_ w420]
                      frame False {
                      }
                      frame True {
                        n230 = call "获取最近两组水样测试数据.vi"("error in (no error)"=w421, "运行模式"=w420, "table"="DO") -> ("error out"=w425:errorcluster, "存储变量"=w424:T16)  [unwired: 7 in]
                        n231 = call "集成干预测试数据存储.vi"("error in (no error)"=w425, "存储变量"=w424) -> ("error out"=w422:errorcluster)  [unwired: 9 in]
                      }
                    }
                    n232 = global read "断电保存变量.vi" "Cond"() -> (w386:bool)
                    n233 = case shown="真" w386 {
                      tunnel: [_ w416] -> w392
                      tunnel: w393 -> [_ w415]
                      tunnel: w382 -> [_ w414]
                      frame False {
                      }
                      frame True {
                        n234 = call "获取最近两组水样测试数据.vi"("error in (no error)"=w415, "运行模式"=w414, "table"="电导率") -> ("error out"=w419:errorcluster, "存储变量"=w418:T16)  [unwired: 7 in]
                        n235 = call "集成干预测试数据存储.vi"("error in (no error)"=w419, "存储变量"=w418) -> ("error out"=w416:errorcluster)  [unwired: 9 in]
                      }
                    }
                    n236 = global read "断电保存变量.vi" "Turb"() -> (w385:bool)
                    n237 = case shown="真" w385 {
                      tunnel: [_ w410] -> w391
                      tunnel: w392 -> [_ w409]
                      tunnel: w382 -> [_ w408]
                      frame False {
                      }
                      frame True {
                        n238 = call "获取最近两组水样测试数据.vi"("error in (no error)"=w409, "运行模式"=w408, "table"="浊度") -> ("error out"=w413:errorcluster, "存储变量"=w412:T16)  [unwired: 7 in]
                        n239 = call "集成干预测试数据存储.vi"("error in (no error)"=w413, "存储变量"=w412) -> ("error out"=w410:errorcluster)  [unwired: 9 in]
                      }
                    }
                    n240 = global read "断电保存变量.vi" "叶绿素a启用"() -> (w384:bool)
                    n241 = case shown="真" w384 {
                      tunnel: [_ w404] -> w390
                      tunnel: w391 -> [_ w403]
                      tunnel: w382 -> [_ w402]
                      frame False {
                      }
                      frame True {
                        n242 = call "获取最近两组水样测试数据.vi"("error in (no error)"=w403, "运行模式"=w402, "table"="叶绿素a") -> ("error out"=w407:errorcluster, "存储变量"=w406:T16)  [unwired: 7 in]
                        n243 = call "集成干预测试数据存储.vi"("error in (no error)"=w407, "存储变量"=w406) -> ("error out"=w404:errorcluster)  [unwired: 9 in]
                      }
                    }
                    n244 = global read "断电保存变量.vi" "藻密度"() -> (w383:bool)
                    n245 = case shown="真" w383 {
                      tunnel: [_ w398] -> _
                      tunnel: w390 -> [_ w397]
                      tunnel: w382 -> [_ w396]
                      frame False {
                      }
                      frame True {
                        n246 = call "获取最近两组水样测试数据.vi"("error in (no error)"=w397, "运行模式"=w396, "table"="藻密度") -> ("error out"=w401:errorcluster, "存储变量"=w400:T16)  [unwired: 7 in]
                        n247 = call "集成干预测试数据存储.vi"("error in (no error)"=w401, "存储变量"=w400) -> ("error out"=w398:errorcluster)  [unwired: 9 in]
                      }
                    }
                  }
                }
              }
            }
          }
        }
        n248 = Unbundle By Name(w242) -> ("R0"=w241:i16)
        n249 = Equal To 0?(x=w241) -> (x = 0?=w240:bool)
        n250 = Select(t=enum16{"初始化", "采配水启动", "仪器操作", "反冲洗", "结束"}."结束" ("枚举"), s=w240, f=enum16{"初始化", "采配水启动", "仪器操作", "反冲洗", "结束"}."反冲洗" ("枚举")) -> (s? t:f=w237:enum16{"初始化", "采配水启动", "仪器操作", "反冲洗", "结束"})
      }
      frame "结束" {
        n251 = Release Queue(queue=w453) -> ()  [unwired: 2 in, 3 out]
        n252 = Unbundle By Name(w450) -> ("测试模式"=w451:enum16{"正常测试", "集成干预"})
        n253 = Cancel Notification(0:w454) -> (8:w455:refnum<notifier>)  [unwired: 1 in, 2 out]
        n254 = case shown="\"集成干预\"" w451 {
          tunnel: w449 -> [_ w458]
          frame "正常测试", Default {
          }
          frame "集成干预" {
            n255 = global write "系统设置全局变量.vi" "运行模式"(w458) -> ()
          }
        }
        n256 = Release Notifier(notifier=w455) -> ()  [unwired: 2 in, 3 out]
      }
    }
    n257 = Wait (ms)(milliseconds to wait=u32 1000 ("等待时间（毫秒）")) -> ()  [unwired: 1 out]
    n258 = Format Into String(format string="%s,当前运行时间%d秒" ("格式字符串"), w15, w11) -> (resulting string=w16:string)  [unwired: 2 in, 1 out]
    n259 = global write "采配水全局变量.vi" "运行状态显示"(w16) -> ()
  }
